vi "PID_screen_V1.2.vi"() -> ()   [LabVIEW 2022 SP3]
panel:
  out "Countdown Timer (CDT)":dbl format="T%<+%H:%M:%S%3u>t"
  out "Date":timestamp format="%<%d/%m/%Y>T"
  in  "Close":bool
  in  "Screen No":dbl
  out "Indian Standard Time (IST)":timestamp format="%<%H:%M:%S%2u>T"
  out "B_GN_PV_07_HSS":bool
  out "B_GN_PV_07":bool
  out "B_GN_PV_02_HSS":bool
  out "B_GN_PV_02":bool
  out "B_LO_P_08":dbl format="%.2f bar"
  out "B_LO_PV_09_HSS":bool
  out "B_LO_PV_09":bool
  out "B_LO_PV_13":bool
  out "B_LO_PV_13_HSS":bool
  out "B_LN_T_03":dbl format="%.2f bar"
  out "B_LO_PV_08":bool
  out "B_LO_PV_08_HSS":bool
  out "B_LO_P_03":dbl format="%.2f bar"
  out "B_LO_T_03":dbl format="%.2f bar"
  out "B_LO_P_09":dbl format="%.2f bar"
  out "B_LO_PV_07":bool
  out "B_LO_PV_07_HSS":bool
  out "B_LO_PV_04":bool
  out "B_LO_PV_04_HSS":bool
  out "B_LO_P_10":dbl format="%.2f bar"
  out "B_LN_P_08":dbl format="%.2f bar"
  out "B_LO_T_05":dbl format="%.2f bar"
  out "B_LO_P_05":dbl format="%.2f bar"
  out "B_LO_T_04":dbl format="%.2f bar"
  out "B_LO_P_04":dbl format="%.2f bar"
  out "B_LO_PV_06":bool
  out "B_LO_PV_06_HSS":bool
  out "B_LO_PV_05":bool
  out "B_LO_PV_05_HSS":bool
  out "LOX_31KL_Tank":dbl(slide) scale=0.0..300.0
  out "B_LO_T_06":dbl format="%.2f bar"
  out "B_LO_P_06":dbl format="%.2f bar"
  out "P_GN_PV_09":bool
  out "P_GN_PV_09_HSS":bool
  out "P_GN_PV_08":bool
  out "P_GN_PV_08_HSS":bool
  out "B_LO_PV_10":bool
  out "B_LO_PV_10_HSS":bool
  out "B_LO_PV_12":bool
  out "B_LO_PV_12_HSS":bool
  out "B_LO_PV_11":bool
  out "B_LO_PV_11_HSS":bool
  out "B_LO_PV_03":bool
  out "B_LO_PV_03_HSS":bool
  out "B_LO_PV_02":bool
  out "B_LO_PV_02_HSS":bool
  out "B_GN_PV_03":bool
  out "B_GN_PV_03_HSS":bool
  out "B_LO_T_02":dbl format="%.2f bar"
  out "B_LO_P_02":dbl format="%.2f bar"
  out "B_GO_P_02":dbl format="%.2f bar"
  out "B_GO_P_01":dbl format="%.2f bar"
  out "B_GN_P_12":dbl format="%.2f bar"
  out "B_GN_T_01":dbl format="%.2f bar"
  out "B_GN_P_11":dbl format="%.2f bar"
  out "B_HE_P_04":dbl format="%.2f bar"
  out "B_HE_T_03":dbl format="%.2f bar"
  out "B_HE_P_03":dbl format="%.2f bar"
  out "B_HE_T_02":dbl format="%.2f bar"
  out "B_HE_P_02":dbl format="%.2f bar"
  out "B_HE_P_01":dbl format="%.2f bar"
  out "B_HE_T_01":dbl format="%.2f bar"
  out "B_LO_P_11":dbl format="%.2f bar"
  out "B_LO_P_07":dbl format="%.2f bar"
  out "B_LO_PV_01_HSS":bool
  out "B_LO_PV_01":bool
  out "B_GN_PV_04_HSS":bool
  out "B_GN_PV_04":bool
  out "B_LO_T_01":dbl format="%.2f bar"
  out "B_LO_P_01":dbl format="%.2f bar"
  out "B_GN_P_33":dbl format="%.2f bar"
  out "B_GN_P_32":dbl format="%.2f bar"
  out "GOX_Tank":u16(slide) scale=0.0..100.0
  out "B_GN_P_10":dbl format="%.2f bar"
  out "B_GN_P_09":dbl format="%.2f bar"
  out "B_GN_P_08":dbl format="%.2f bar"
  out "B_GN_P_07":dbl format="%.2f bar"
  out "B_GN_P_06":dbl format="%.2f bar"
  out "B_GN_P_05":dbl format="%.2f bar"
  out "B_GN_P_04":dbl format="%.2f bar"
  out "B_GN_P_03":dbl format="%.2f bar"
  out "B_GN_P_02":dbl format="%.2f bar"
  out "B_GN_P_01":dbl format="%.2f bar"
  out "B_GO_P_04":dbl format="%.2f bar"
  out "B_GN_P_13":dbl format="%.2f bar"
  out "B_GO_P_03":dbl format="%.2f bar"
  out "B_GN_CV_01":bool caption="Boolean"
  # "BSTF PID SCREEN"
  # "VERSION 1.1"
  # "Connected to\nStage COPV \nUbmilical"
  # "To Atmosphere"
  # "To Atmosphere"
  # "To Atmosphere"
  # "LOX/LIN Ground Valves Command"
  # "Stage Cryo Valves Command"
  # "To Atmosphere"
  # "LOX Tank Pressurization"
  # "B_GN_CV_01"
  # "GOX Ignitor Purge"
  # "LOX/LIN Feed Line Purge"
  # "Engine LOX Injector Purge"
  # "To Atmosphere"
  # "To Atmosphere"
  # "Connect to all ground\nLOX and LIN EV"
  # "Connect to all stage\nLOX and LIN EV"
  # "LOX Tank\nVent"
  # "B_LO_SP_01"
  # "ENGINE"
  # "LOX CLUSTER MANIFOLD"
  # "TO STAGE FILL/DRAIN"
  # "GOX IGNITOR PURGE"
  # "B_GN_PV_07"
  # "B_GN_PV_02"
  # "B_LO_PV_09"
  # "B_LO_PV_13"
  # "B_LO_PV_08"
  # "B_LO_PV_07"
  # "B_LO_PV_04"
  # "B_LO_PV_06"
  # "B_LO_PV_05"
  # "LOX\n31KL\nTANK"
  # "P_GN_PV_09"
  # "P_GN_PV_08"
  # "B_LO_PV_10"
  # "B_LO_PV_12"
  # "B_LO_PV_11"
  # "B_LO_PV_03"
  # "B_LO_PV_02"
  # "B_GN_PV_03"
  # "LOX\nFILL"
  # "STAGE SUBCOOL RETURN"
  # "B_LO_PV_01"
  # "B_GN_PV_04"
  # "GN2"
  # "GOX MANIFOLD"
  # "GN2"
  # "GOX"
  # "GN2"
  # "GN2"
  # "GN2"
  # "GN2"
  # "GN2"
  # "LOX PUMP SEAL PURGE"
  # "Common\nGN2\nSource"
  # "GOX\nSource"
  # "BOOSTER PUMP"
  # "GHe\nSource"
  # "GN2\nVaporiser/\nSource"
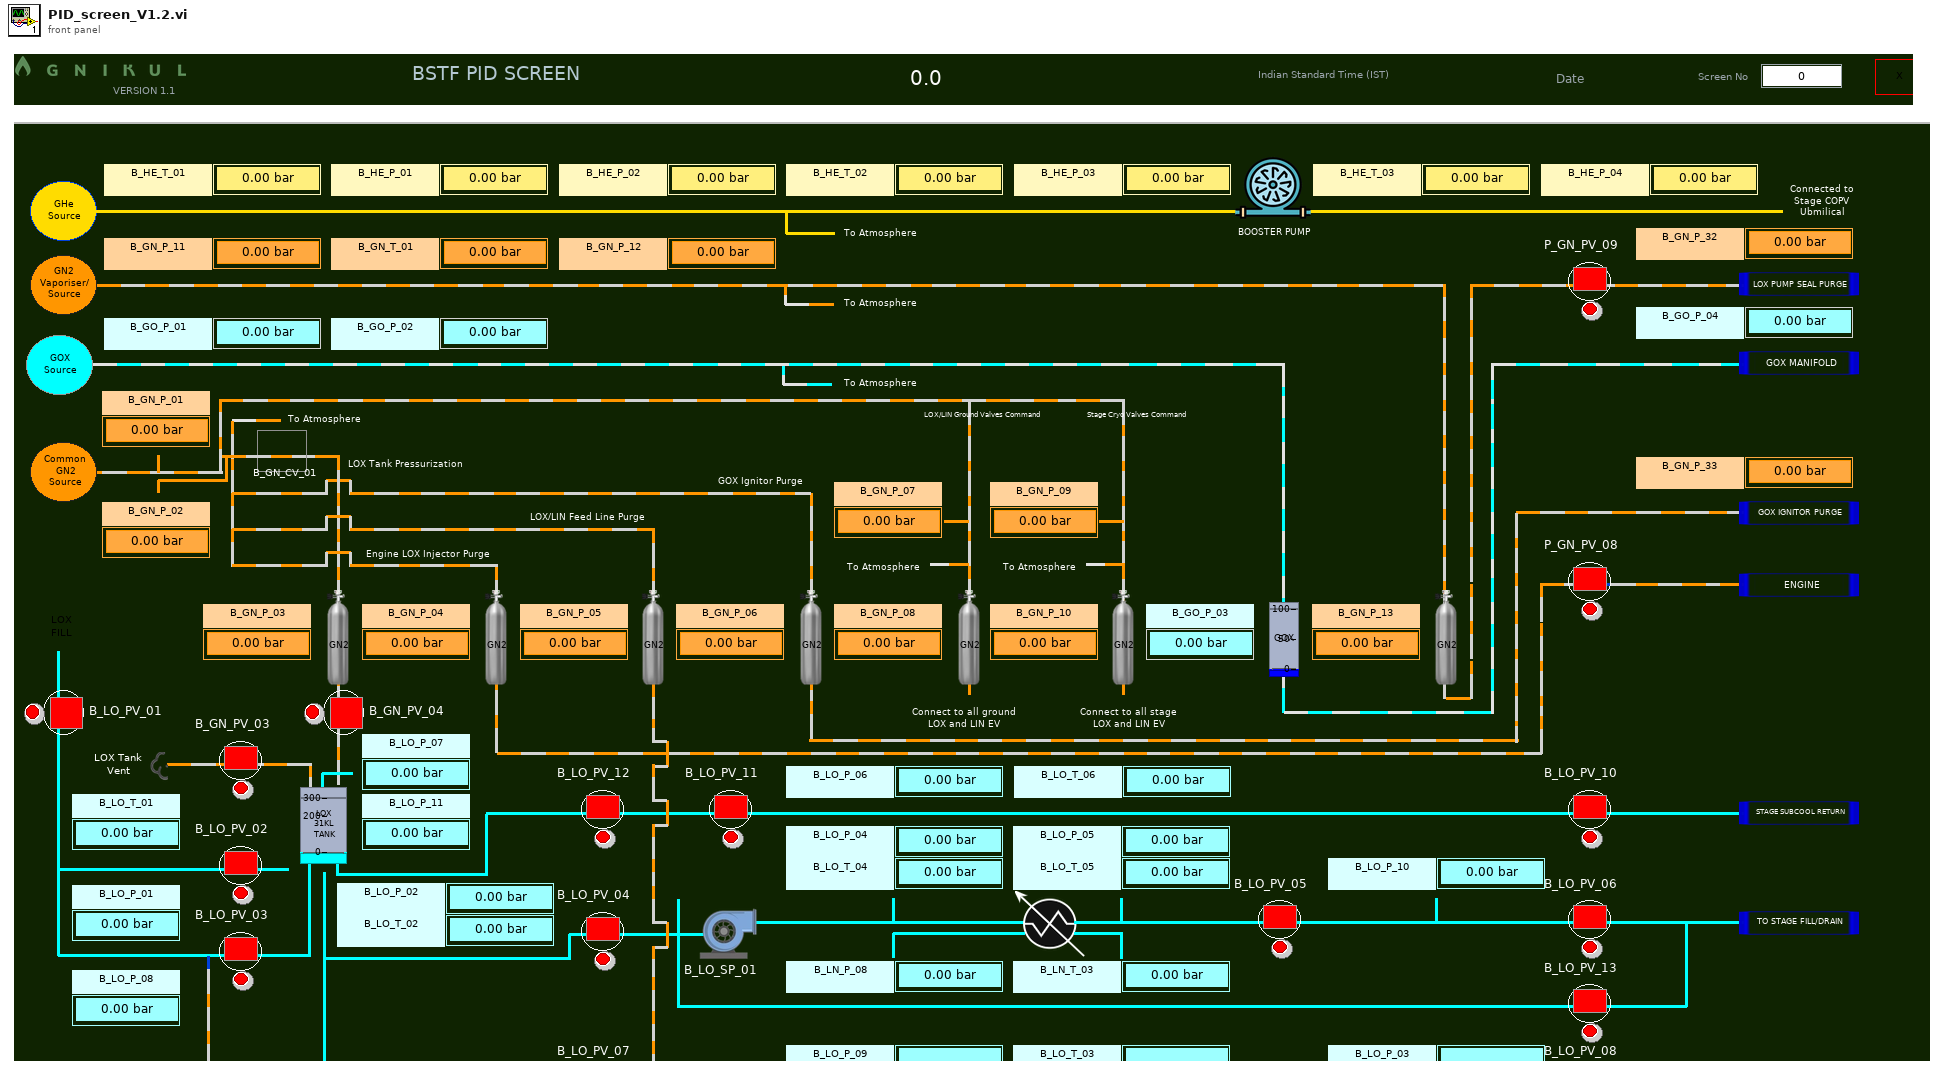
[diagram p1: front panel]
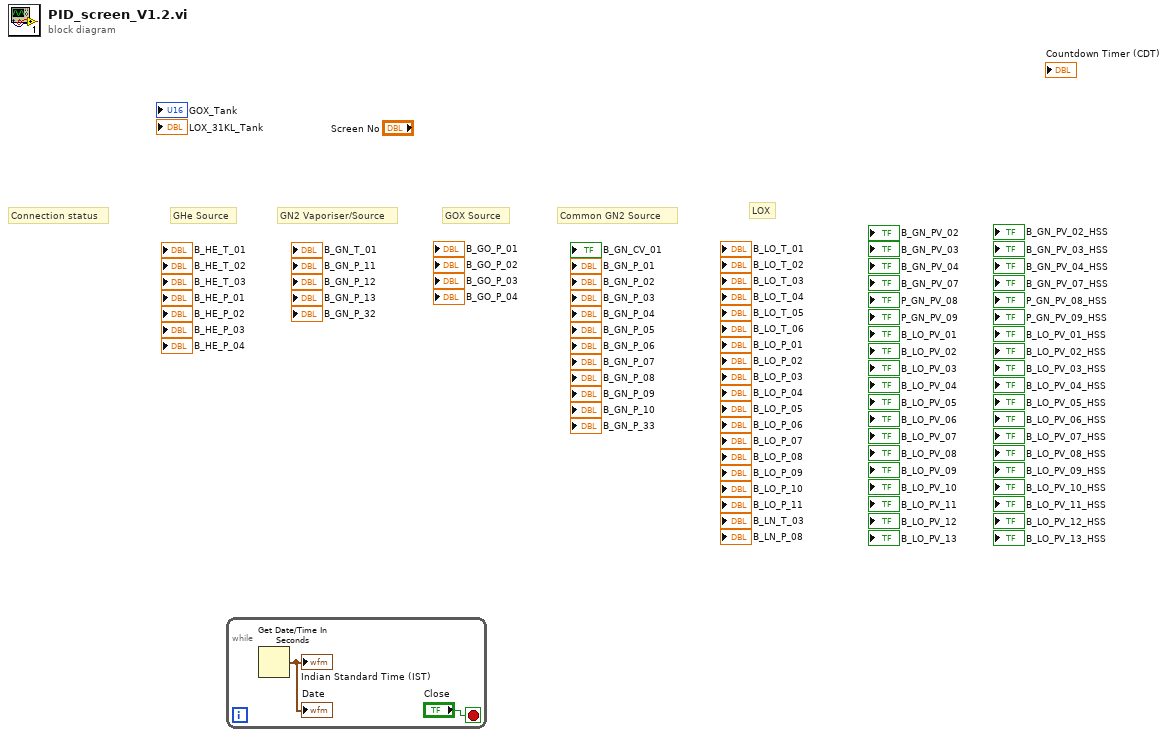
[diagram p0: block diagram]
diagram:
  # "Connection status"
  # "LOX"
  # "Common GN2 Source"
  # "GOX Source"
  # "GN2 Vaporiser/Source"
  # "GHe Source"
  n1 = while {
    stop <- "Close" stop-if-true
    n2 = Get Date/Time In Seconds() -> (seconds since 1Jan1904=→"Indian Standard Time (IST)" →"Date":timestamp)
  }
